vi "SDecoder.vi"(8 "error in (no error)":errorcluster, 11 "Input String":string) -> (0 "error out":errorcluster, 1 "Measured Volts":dbl format="%.2f", 2 "Blue On?":bool, 3 "Green On?":bool)   [LabVIEW 2018]
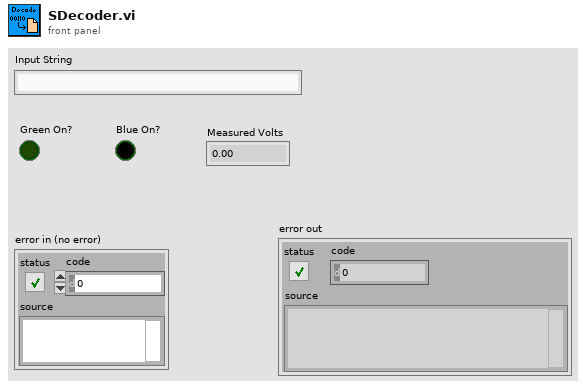
[diagram p1: front panel]
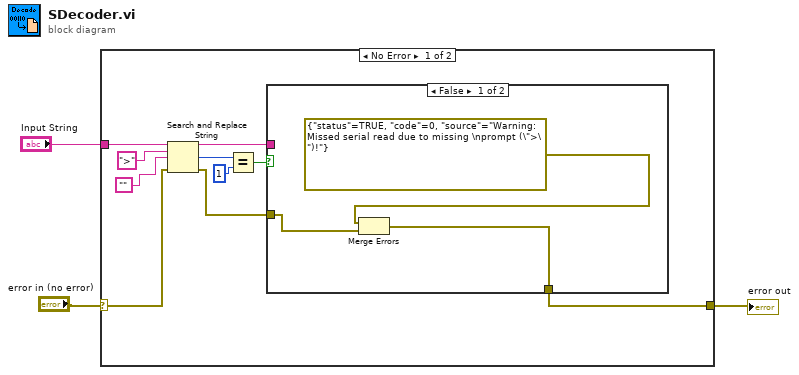
[diagram p0: block diagram]
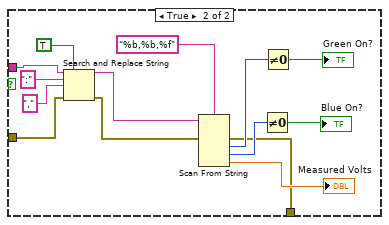
[diagram p2: hidden frame]
diagram:
  n1 = case shown="No Error" "error in (no error)" {
    selector: "error in (no error)" -> [w11 w31]
    tunnel: "Input String" -> [w13 _]
    tunnel: [w5 w31] -> w1
    frame No Error {
      n2 = Search and Replace String(input string=w13, search string=">", replace string="", error in=w11) -> (result string=w7:string, number of replacements=w9:i32, error out=w6:errorcluster)  [unwired: 4 in, 1 out]
      n3 = Equal?(x=w9, y=1) -> (x = y?=w8:bool)
      n4 = case shown="False" w8 {
        tunnel: w7 -> [_ w18]
        tunnel: w6 -> [w16 w22]
        tunnel: [w15 w24] -> w5
        frame False {
          n5 = Merge Errors(errorcluster {"status"=TRUE, "code"=0, "source"="Warning: Missed serial read due to missing \nprompt (\">\")!"} ("error constant"), w16) -> (w15:errorcluster)
        }
        frame True {
          n6 = Search and Replace String(replace all?=TRUE, input string=w18, search string=":", replace string=",", error in=w22) -> (result string=w23:string, error out=w21:errorcluster)  [unwired: 3 in, 2 out]
          n7 = Scan From String(format string="%b,%b,%f", input string=w23, error in=w21) -> (error out=w24:errorcluster, output 1=w25:i32, output 2=w26:i32, output 3=→"Measured Volts":dbl)  [unwired: 4 in, 2 out]
          n8 = Not Equal To 0?(x=w26) -> (x != 0?=→"Blue On?":bool)
          n9 = Not Equal To 0?(x=w25) -> (x != 0?=→"Green On?":bool)
        }
      }
    }
    frame Error {
    }
  }
  "error out" <- w1
